vi "Handle Overlays.vi"(8 "error in (no error)":errorcluster, 9 "Overlays":refnum<class "Config Storage.lvclass">[](array[class]), 10 "Config":refnum<class "Config Manager.lvclass">, 11 "Config Storage in":refnum<class "Config Storage.lvclass">) -> (0 "error out":errorcluster, 3 "Config Storage out":refnum<class "Config Storage.lvclass">)   [LabVIEW 2020, in "CDM-Config.lvlib" / "Config Storage.lvclass"]
uses:
  Config Storage.lvclass
  Config Manager/Config Manager.lvclass
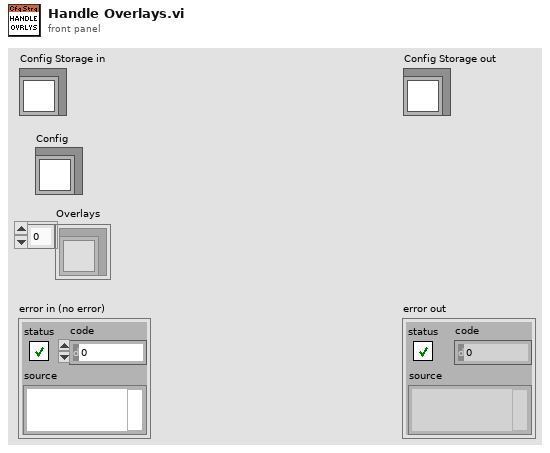
[diagram p1: front panel]
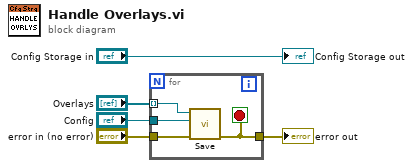
[diagram p0: block diagram]
diagram:
  n1 = for {
    tunnel: "error in (no error)" -> [w9]
    tunnel: "Overlays" -> [w7] mode=indexing
    tunnel: "Config" -> [w8]
    tunnel: [w6] -> w1
    stop <- w6 stop-if-true
    n2 = call "Save.vi"("error in (no error)"=w9, "Config"=w8, "Config Storage in"=w7) -> ("error out"=w6:errorcluster)  [unwired: 7 in, 1 out]
  }
  "error out" <- w1
  "Config Storage out" <- "Config Storage in"
